vi "FlexDDS-NG_DCP_Sweep.vi"(5 "f1":dbl=30000000.0, 6 "jump before ramp":bool, 7 "f0":dbl=45000000.0, 8 "sweep time tolerance (us)":dbl=0.01, 9 "sweep time (ms)":dbl=2000.0, 10 "Channels in":T1(ring), 11 "initial instruction string":string) -> (3 "appended instruction string out":string)   [LabVIEW 2016]
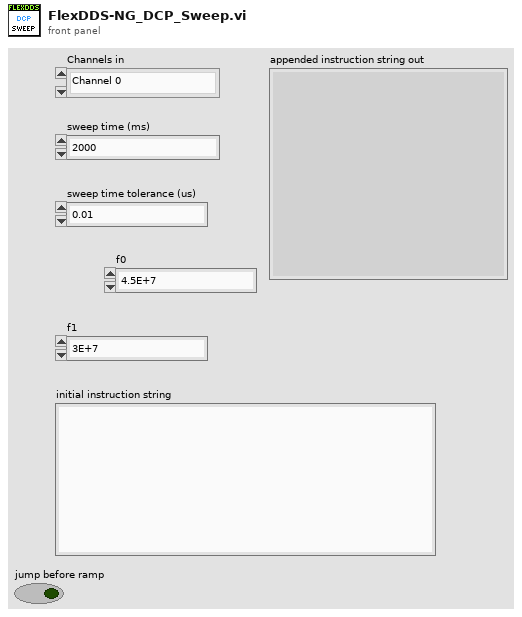
[diagram p1: front panel]
types:
  T1 = enum32{"Channel 0", "Channel 1", "Both channels"}
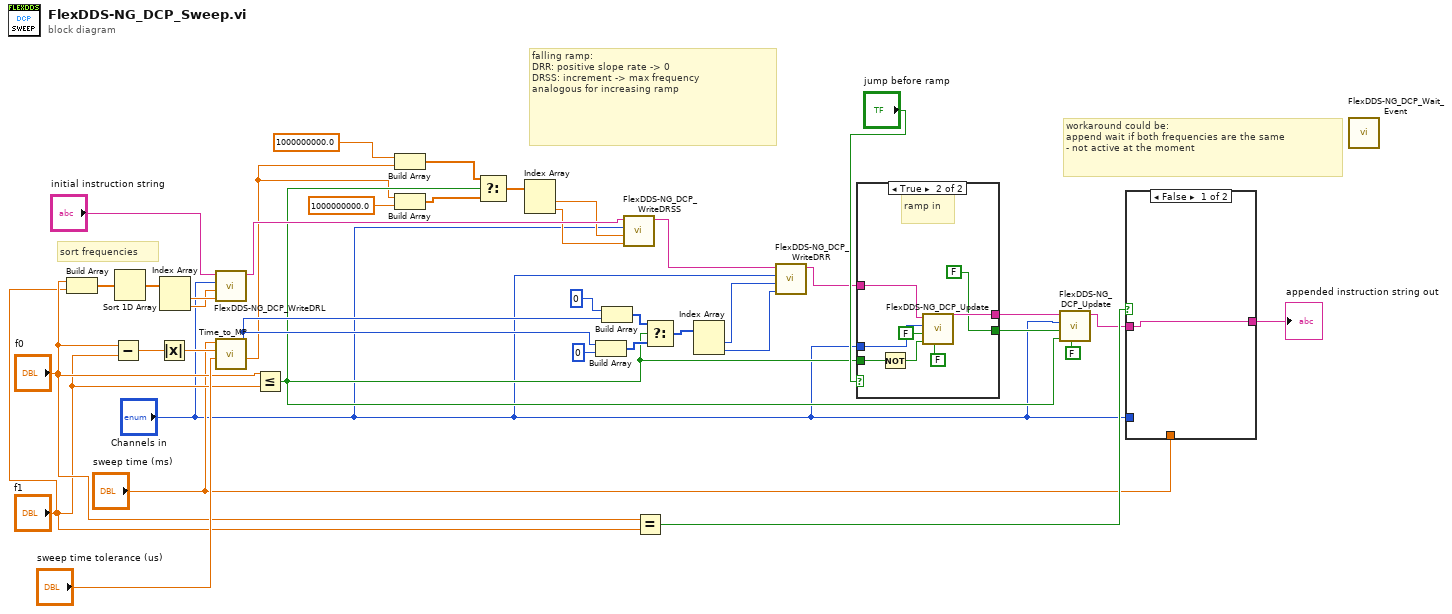
[diagram p0: block diagram]
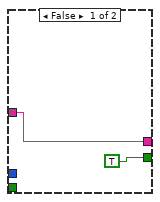
[diagram p3: hidden frame]
diagram:
  # "workaround could be:\nappend wait if both frequencies are the same\n- not active at the moment"
  # "falling ramp:\nDRR: positive slope rate -> 0\nDRSS: increment -> max frequency\nanalogous for increasing ramp"
  # "sort frequencies"
  n1 = Build Array("f0", "f1") -> (w35:dbl[])
  n2 = Subtract(x="f0", y="f1") -> (x-y=w33:dbl)
  n3 = Sort 1D Array(array=w35) -> (sorted array=w36:dbl[])
  n4 = Absolute Value(x=w33) -> (abs(x)=w34:dbl)
  n5 = Index Array(array=w36) -> (element #1=w38:dbl, element #2=w37:dbl)  [unwired: 2 in]
  n6 = call "FlexDDS-NG_DCP_WriteDRL.vi"("low limit"=w38, "high limit"=w37, "Channels"="Channels in", "initial instruction string"="initial instruction string") -> ("appended instruction string"=w31:string)  [unwired: 7 in]
  n7 = call "Time_to_MP.vi"("sweep time tolerance (us)"="sweep time tolerance (us)", "freq_diff (Hz)"=w34, "sweep time (ms)"="sweep time (ms)") -> ("Dt"=w17:dbl, "P"=w21:u32)  [unwired: 2 in, 5 out]
  n8 = Less Or Equal?(x="f0", y="f1") -> (x <= y?=w18:bool)
  n9 = Build Array(1000000000.0 ("element"), w17) -> (w14:dbl[])
  n10 = Build Array(w17, 1000000000.0 ("element")) -> (w13:dbl[])
  n11 = Select(t=w14, s=w18, f=w13) -> (s? t:f=w12:dbl[])
  n12 = Index Array(array=w12) -> (element #1=w11:dbl, element #2=w10:dbl)  [unwired: 2 in]
  n13 = Build Array(w21, u16 0 ("element")) -> (w29:u32[])
  n14 = Build Array(u16 0 ("element"), w21) -> (w28:u32[])
  n15 = call "FlexDDS-NG_DCP_WriteDRSS.vi"("increment step size"=w10, "decrement step size"=w11, "Channels"="Channels in", "initial instruction string"=w31) -> ("appended instruction string"=w30:string)  [unwired: 7 in]
  n16 = Equal?(x="f0", y="f1") -> (x = y?=w5:bool)
  n17 = Select(t=w28, s=w18, f=w29) -> (s? t:f=w27:u32[])
  n18 = Index Array(array=w27) -> (element #1=w26:u32, element #2=w25:u32)  [unwired: 2 in]
  n19 = call "FlexDDS-NG_DCP_WriteDRR.vi"("digital ramp positive slope rate"=w25, "digital ramp negative slope rate"=w26, "Channels"="Channels in", "initial instruction string"=w30) -> ("appended instruction string"=w23:string)  [unwired: 7 in]
  n20 = case shown="True" "jump before ramp" {
    tunnel: w23 -> [w41 w48]
    tunnel: [w41 w49] -> w22
    tunnel: "Channels in" -> [_ w47]
    tunnel: w18 -> [_ w45]
    tunnel: [TRUE FALSE ("IO_UPDATE(true=u, false = '')")] -> w8
    frame False {
    }
    frame True {
      # "ramp in"
      n21 = Not(x=w45) -> (.not. x?=w46:bool)
      n22 = call "FlexDDS-NG_DCP_Update.vi"("ONLY IO_UPDATE"=FALSE, "DRCTL(true=+, false=-)"=w46, "IO_UPDATE(true=u, false = '')"=FALSE, "Channels"=w47, "appended instruction string in"=w48) -> ("appended instruction string out"=w49:string)  [unwired: 6 in]
    }
  }
  n23 = call "FlexDDS-NG_DCP_Update.vi"("ONLY IO_UPDATE"=FALSE, "DRCTL(true=+, false=-)"=w18, "IO_UPDATE(true=u, false = '')"=w8, "Channels"="Channels in", "appended instruction string in"=w22) -> ("appended instruction string out"=w4:string)  [unwired: 6 in]
  n24 = case shown="False" w5 {
    tunnel: w4 -> [w50 w51]
    tunnel: [w50 w51] -> w3
    tunnel: "sweep time (ms)" -> [_ _]
    tunnel: "Channels in" -> [_ _]
    frame False {
    }
    frame True {
    }
  }
  "appended instruction string out" <- w3
  n25 = call "FlexDDS-NG_DCP_Wait_Event.vi"() -> ()  [unwired: 11 in, 1 out]
